vi "salLabviewUserEvent.vi"(8 "error in (no error)":errorcluster, 11 "Events":T1) -> (0 "error out":errorcluster, 2 "SAL Labview event handle":cluster{i32, i32, i32, i32, i32}, 3 "Event Registration Refnum":refnum<event-registration>)   [LabVIEW 2016]
uses:
  <vilib>/Utility/error.llb/DialogType.ctl
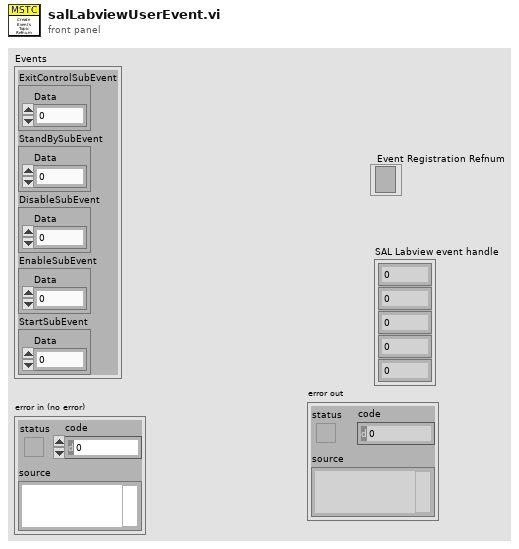
[diagram p1: front panel]
types:
  T1 = cluster{"ExitControlSubEvent":cluster{"Data":i32}, "StandBySubEvent":cluster{"Data":i32}, "DisableSubEvent":cluster{"Data":i32}, "EnableSubEvent":cluster{"Data":i32}, "StartSubEvent":cluster{"Data":i32}}
  T2 = typedef "DialogType.ctl" = u16
  T3 = cluster{"Exit":i32, "Standby":i32, "Disable":i32, "Enable":i32, "Start":i32}
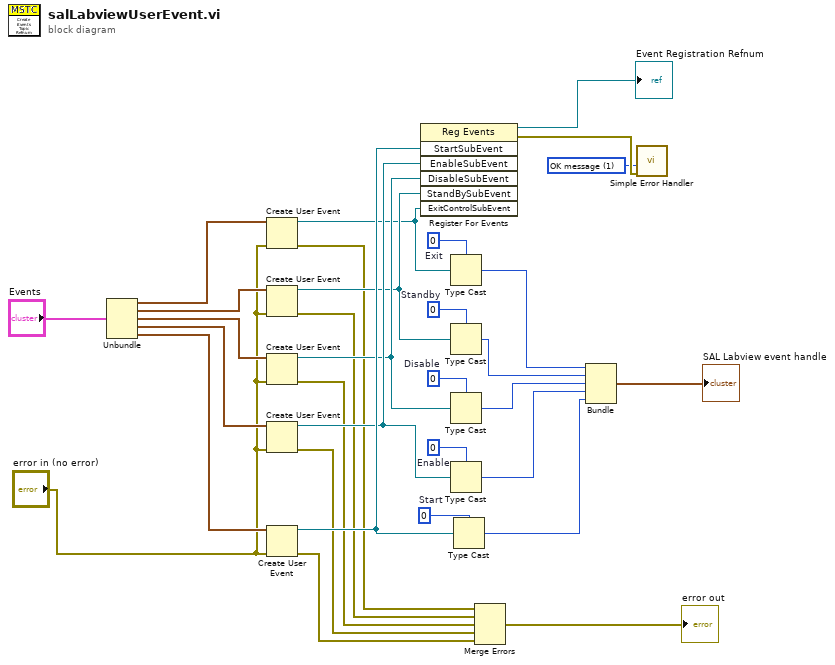
[diagram p0: block diagram]
diagram:
  w24 = 0  # Exit
  w26 = 0  # Standby
  w28 = 0  # Disable
  w30 = 0  # Enable
  w32 = 0  # Start
  w10 = T2 1 items=["no dialog", "OK message", "continue or stop message", "OK message + warnings", "continue/stop + warnings"] ("type of dialog (OK msg:1)")
  n1 = Unbundle("Events") -> ("ExitControlSubEvent"=w16:cluster{"Data":i32}, "StandBySubEvent"=w15:cluster{"Data":i32}, "DisableSubEvent"=w14:cluster{"Data":i32}, "EnableSubEvent"=w13:cluster{"Data":i32}, "StartSubEvent"=w12:cluster{"Data":i32})
  n2 = Create User Event(user event datatype=w16, error in="error in (no error)") -> (user event=w23:refnum<user-event>, error out=w6:errorcluster)
  n3 = Create User Event(user event datatype=w15, error in="error in (no error)") -> (user event=w25:refnum<user-event>, error out=w5:errorcluster)
  n4 = Create User Event(user event datatype=w14, error in="error in (no error)") -> (user event=w27:refnum<user-event>, error out=w4:errorcluster)
  n5 = Create User Event(user event datatype=w13, error in="error in (no error)") -> (user event=w29:refnum<user-event>, error out=w3:errorcluster)
  n6 = Create User Event(user event datatype=w12, error in="error in (no error)") -> (user event=w31:refnum<user-event>, error out=w2:errorcluster)
  n7 = register-events(w31, w29, w27, w25, w23) -> (reference out=→"Event Registration Refnum":refnum<event-registration>, error out=w11:errorcluster)  [unwired: 2 in]
  n8 = Type Cast ("Exit")(type=w24, x=w23) -> (*(type *) &x=w21:i32)
  n9 = Type Cast ("Standby")(type=w26, x=w25) -> (*(type *) &x=w20:i32)
  n10 = Type Cast ("Disable")(type=w28, x=w27) -> (*(type *) &x=w17:i32)
  n11 = Type Cast ("Enable")(type=w30, x=w29) -> (*(type *) &x=w18:i32)
  n12 = Type Cast ("Start")(type=w32, x=w31) -> (*(type *) &x=w19:i32)
  n13 = Merge Errors(w6, w5, w4, w3, w2) -> (→"error out":errorcluster)
  n14 = Bundle("Exit"=w21, "Standby"=w20, "Disable"=w17, "Enable"=w18, "Start"=w19) -> (→"SAL Labview event handle":T3)  [unwired: 1 in]
  n15 = call <vilib>:"Simple Error Handler.vi"("type of dialog (OK msg:1)"=w10, "error in (no error)"=w11) -> ()  [unwired: 3 in, 5 out]
